vi "populateEventForceActuatorInfo.vi"(8 "error in (no error)":errorcluster, 11 "Model in":refnum<class "Model.lvclass">) -> (0 "error out":errorcluster, 3 "Model out":refnum<class "Model.lvclass">)   [LabVIEW 2016, in "Model.lvclass"]
uses:
  Model.lvclass
  Model.lvclass/Model.ctl
  ILCCommunications/ILCCommunications.lvclass/ILCCommunications.ctl
  Publisher/Publisher.lvclass/Publisher.ctl
  Common_RT_FAILC/FAILC/FAILC.lvclass/FAILC.ctl
  Common_RT_ILC/ILC/ILC.lvclass/ILC.ctl
  Common_RT_FAILC/FAILC/FAILC.lvclass
  D:/Code/ts_M1M3Support/Common_RT_ILC/ILC/ILC.lvclass
  Common_RT_ILC/ILC/ILC.lvclass
  ILCCommunications/ILCCommunications.lvclass
  Publisher/Publisher.lvclass
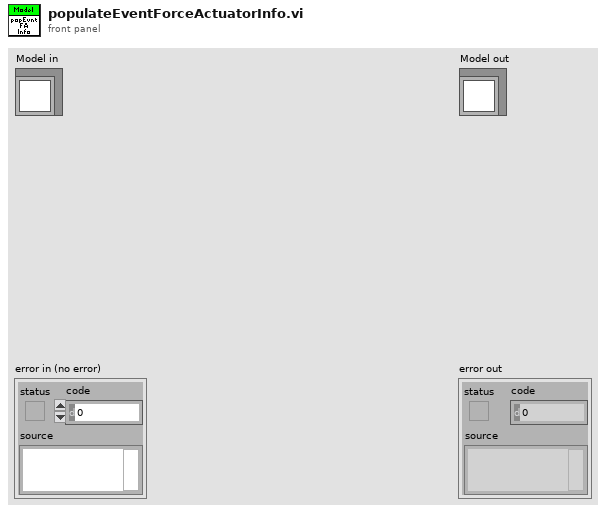
[diagram p1: front panel]
types:
  T1 = typedef "RTILC.lvlib/ILCData.ctl" = cluster{"Constants":T2, "Command":T3, "Telemetry":T5, "Responses":T6, "Timestamps":T8, "Timings":T9}
  T2 = typedef "RTILC.lvlib/ILCConstants.ctl" = cluster{"Subnet":u8, "Address":u8}
  T3 = typedef "RTILC.lvlib/ILCCommand.ctl" = cluster{"Mode":u16, "TemporaryAddress":u8, "ADCScanRate":T4, "ADCChannel":u8, "ADCOffset":sgl, "ADCSensitivity":sgl}
  T4 = typedef "RTILC.lvlib/ILCScanRates.ctl" = u8
  T5 = typedef "RTILC.lvlib/ILCTelemetry.ctl" = cluster{"UniqueID":u64, "FirmwareType":u8, "NetworkNodeType":u8, "ILCOption":u8, "NetworkNodeOption":u8, "MajorRevision":u8, "MinorRevision":u8, "FirmwareName":string, "Mode":u16, "MajorFault":bool, "MinorFault":bool, "FaultOverride":bool, "MainCalibrationError":bool, "BackupCalibrationError":bool, "UniqueIDCRCMismatch":bool, "AppTypeNodeTypeMismatch":bool, "AppMissing":bool, "AppCRCMismatch":bool, "TEDSNotFound":bool, "TEDS1Mismatch":bool, "TEDS2Mismatch":bool, "WatchdogResetDetected":bool, "BrownoutDetected":bool, "EventTrapResetDetected":bool, "MotorPowerFault":bool, "SSRPowerFault":bool, "AuxPowerFault":bool, "SMCPowerFault":bool, "TemporaryAddress":u8, "ADCScanRate":T4, "MainADCCalibrationK":sgl[], "MainSensorOffset":sgl[], "MainSensorSensitivity":sgl[], "BackupADCCalibrationK":sgl[], "BackupSensorOffset":sgl[], "BackupSensorSensitivity":sgl[]}
  T6 = typedef "RTILC.lvlib/ILCResponses.ctl" = cluster{"ReportServerID":T7, "ReportServerStatus":T7, "Mode":T7, "TemporaryAddress":T7, "Reset":T7, "ADCScanRate":T7, "ADCOffsetSensitivity":T7, "ReportCalibrationData":T7}
  T7 = typedef "RTModbus.lvlib/ExceptionCodes.ctl" = u16
  T8 = typedef "RTILC.lvlib/ILCTimestamps.ctl" = cluster{"ReportServerID":dbl, "ReportServerStatus":dbl, "Mode":dbl, "TemporaryAddress":dbl, "Reset":dbl, "ADCScanRate":dbl, "ADCOffsetSensitivity":dbl, "ReportCalibrationData":dbl}
  T9 = typedef "RTILC.lvlib/ILCTimings.ctl" = cluster{"ReportServerID":u32, "ReportServerStatus":u32, "Mode":u32, "TemporaryAddress":u32, "Reset":u32, "ADCScanRate":u32, "ADCOffsetSensitivity":u32, "ReportCalibrationData":u32}
  T10 = typedef "RTFAILC.lvlib/FAData.ctl" = cluster{"Constants":T11, "Command":T13, "Telemetry":T14, "Responses":T15, "Timings":T16, "Timestamps":T17}
  T11 = typedef "RTFAILC.lvlib/FAConstants.ctl" = cluster{"ID":i16, "Type":T12, "XPosition":sgl, "YPosition":sgl, "ZPosition":sgl}
  T12 = typedef "RTFAILC.lvlib/FATypes.ctl" = enum16{"SingleAxis", "DualAxis"}
  T13 = typedef "RTFAILC.lvlib/FACommand.ctl" = cluster{"AxialSetPoint":i32, "LateralSetPoint":i32, "AxialBoosterValveGain":sgl, "LateralBoosterValveGain":sgl}
  T14 = typedef "RTFAILC.lvlib/FATelemetry.ctl" = cluster{"ILCFault":bool, "DCAFault":bool, "BroadcastCounter":u8, "AxialLoadCellForce":sgl, "LateralLoadCellForce":sgl, "AxialBoosterValveGain":sgl, "LateralBoosterValveGain":sgl}
  T15 = typedef "RTFAILC.lvlib/FAResponses.ctl" = cluster{"BoosterValveGain":T7, "ReadBoosterValveGain":T7, "SetForce":T7, "ForceAndStatus":T7}
  T16 = typedef "RTFAILC.lvlib/FATimings.ctl" = cluster{"BroadcastSetForce":u32, "BoosterValveGain":u32, "FreezeSensorValues":u32, "ForceAndStatus":u32, "ReadBoosterValveGain":u32, "SetForce":u32}
  T17 = typedef "RTFAILC.lvlib/FATimestamps.ctl" = cluster{"BroadcastSetForce":dbl, "BoosterValveGain":dbl, "FreezeSensorValues":dbl, "ForceAndStatus":dbl, "ReadBoosterValveGain":dbl, "SetForce":dbl}
  T18 = typedef "M1M3SupportTopics.lvlib/Timestamp.ctl" = dbl
  T19 = typedef "M1M3SupportTopics.lvlib/EventForceActuatorInfo.ctl" = cluster{"Timestamp":T18, "ReferenceId":i32[], "XPosition":sgl[], "YPosition":sgl[], "ZPosition":sgl[], "ILCUniqueId":i64[], "ILCApplicationType":u8[], "NetworkNodeType":u8[], "ILCSelectedOptions":u8[], "NetworkNodeOptions":u8[], "MajorRevision":u8[], "MinorRevision":u8[], "ADCScanRate":u8[], "MainADCCalibrationK1":sgl[], "MainADCCalibrationK2":sgl[], "MainADCCalibrationK3":sgl[], "MainADCCalibrationK4":sgl[], "MainAxialLoadCellOffset":sgl[], "MainLateralLoadCellOffset":sgl[], "MainAxialLoadCellSensitivity":sgl[], "MainLateralLoadCellSensitivity":sgl[], "BackupADCCalibrationK1":sgl[], "BackupADCCalibrationK2":sgl[], "BackupADCCalibrationK3":sgl[], "BackupADCCalibrationK4":sgl[], "BackupAxialLoadCellOffset":sgl[], "BackupLateralLoadCellOffset":sgl[], "BackupAxialLoadCellSensitivity":sgl[], "BackupLateralLoadCellSensitivity":sgl[], "DCAAxialGain":sgl[], "DCALateralGain":sgl[], "DCAUniqueId":i64[], "DCAFirmwareType":u8[], "DCAMajorRevision":u8[], "DCAMinorRevision":u8[], "MainCalibrationError":bool[], "BackupCalibrationError":bool[], "DCAFirmwareUpdate":bool[], "UniqueIdCRCError":bool[], "ApplicationTypeMismatch":bool[], "ApplicationMissing":bool[], "ApplicationCRCMismatch":bool[], "OneWireMissing":bool[], "OneWire1Mismatch":bool[], "OneWire2Mismatch":bool[], "DCAUniqueIdCRCError":bool[], "DCAMainCalibrationError":bool[], "DCABackupCalibrationError":bool[], "DCAApplicationMissing":bool[], "DCAApplicationCRCMismatch":bool[], "DCABootloaderActive":bool[]}
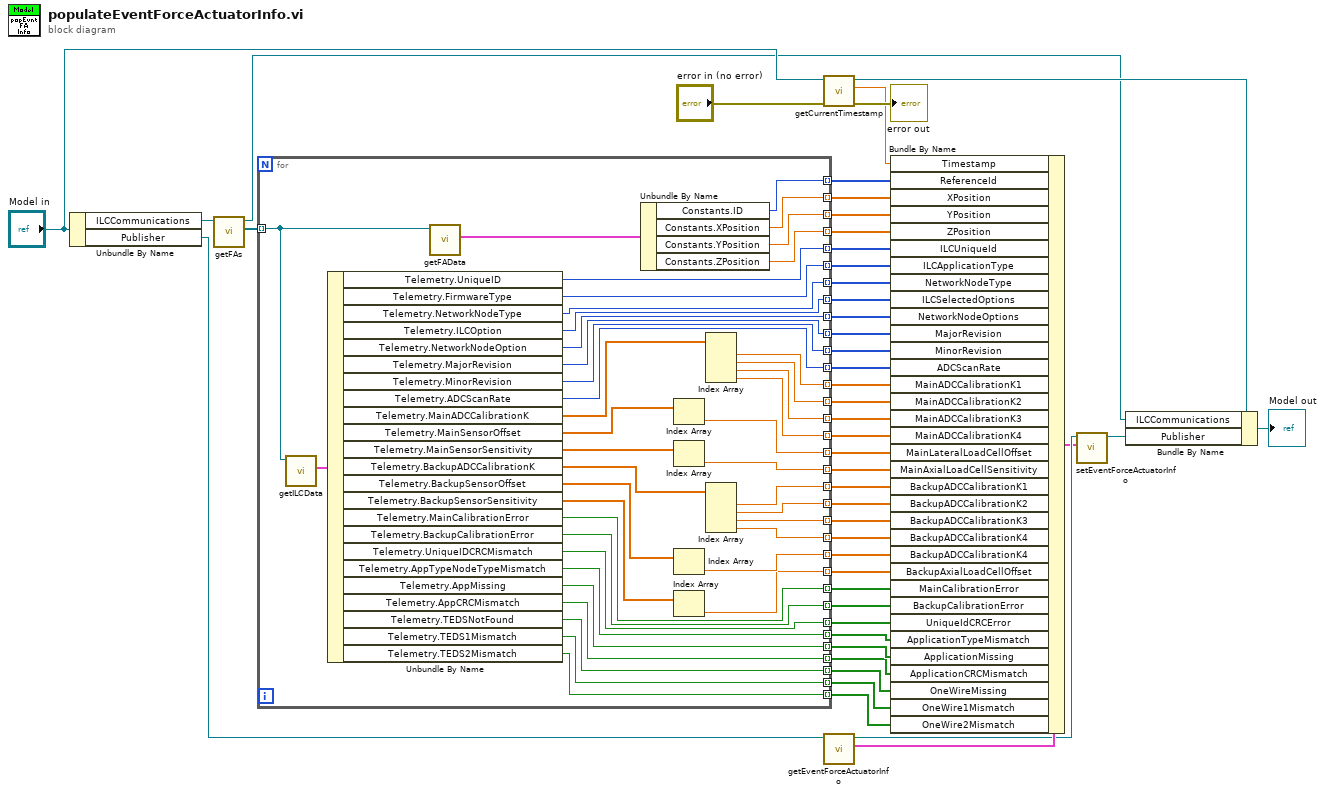
[diagram p0: block diagram]
diagram:
  n1 = Unbundle By Name("Model in") -> ("ILCCommunications"=w8:refnum<class "ILCCommunications.lvclass">, "Publisher"=w5:refnum<class "Publisher.lvclass">)
  n2 = call "getFAs.vi"("ILCCommunications in"=w8) -> ("FAs"=w6:refnum<class "FAILC.lvclass">[], "ILCCommunications out"=w7:refnum<class "ILCCommunications.lvclass">)  [unwired: 9 in]
  n3 = for {
    tunnel: w6 -> [w49] mode=indexing
    tunnel: [w87] -> w46 mode=indexing
    tunnel: [w86] -> w45 mode=indexing
    tunnel: [w85] -> w44 mode=indexing
    tunnel: [w84] -> w43 mode=indexing
    tunnel: [w83] -> w42 mode=indexing
    tunnel: [w82] -> w41 mode=indexing
    tunnel: [w81] -> w40 mode=indexing
    tunnel: [w80] -> w39 mode=indexing
    tunnel: [w79] -> w38 mode=indexing
    tunnel: [w78] -> w37 mode=indexing
    tunnel: [w77] -> w36 mode=indexing
    tunnel: [w76] -> w35 mode=indexing
    tunnel: [w74] -> w34 mode=indexing
    tunnel: [w72] -> w33 mode=indexing
    tunnel: [w70] -> w32 mode=indexing
    tunnel: [w69] -> w31 mode=indexing
    tunnel: [w68] -> w30 mode=indexing
    tunnel: [w67] -> w29 mode=indexing
    tunnel: [w65] -> w28 mode=indexing
    tunnel: [w63] -> w27 mode=indexing
    tunnel: [w62] -> w26 mode=indexing
    tunnel: [w61] -> w25 mode=indexing
    tunnel: [w60] -> w24 mode=indexing
    tunnel: [w59] -> w23 mode=indexing
    tunnel: [w58] -> w22 mode=indexing
    tunnel: [w57] -> w21 mode=indexing
    tunnel: [w56] -> w20 mode=indexing
    tunnel: [w55] -> w19 mode=indexing
    tunnel: [w54] -> w18 mode=indexing
    tunnel: [w53] -> w17 mode=indexing
    tunnel: [w52] -> w11 mode=indexing
    tunnel: [w51] -> w10 mode=indexing
    tunnel: [w50] -> w9 mode=indexing
    n4 = call "getILCData.vi"("ILC in"=w49) -> ("ILCData"=w89:T1)  [unwired: 9 in, 1 out]
    n5 = Unbundle By Name(w89) -> ("Telemetry.UniqueID"=w87:u64, "Telemetry.FirmwareType"=w86:u8, "Telemetry.NetworkNodeType"=w85:u8, "Telemetry.ILCOption"=w84:u8, "Telemetry.NetworkNodeOption"=w83:u8, "Telemetry.MajorRevision"=w82:u8, "Telemetry.MinorRevision"=w81:u8, "Telemetry.ADCScanRate"=w80:T4, "Telemetry.MainADCCalibrationK"=w88:sgl[], "Telemetry.MainSensorOffset"=w75:sgl[], "Telemetry.MainSensorSensitivity"=w73:sgl[], "Telemetry.BackupADCCalibrationK"=w71:sgl[], "Telemetry.BackupSensorOffset"=w66:sgl[], "Telemetry.BackupSensorSensitivity"=w64:sgl[], "Telemetry.MainCalibrationError"=w62:bool, "Telemetry.BackupCalibrationError"=w61:bool, "Telemetry.UniqueIDCRCMismatch"=w60:bool, "Telemetry.AppTypeNodeTypeMismatch"=w59:bool, "Telemetry.AppMissing"=w58:bool, "Telemetry.AppCRCMismatch"=w57:bool, "Telemetry.TEDSNotFound"=w56:bool, "Telemetry.TEDS1Mismatch"=w55:bool, "Telemetry.TEDS2Mismatch"=w54:bool)
    n6 = call "getFAData.vi"("FAILC in"=w49) -> ("FAData"=w48:T10)  [unwired: 9 in, 1 out]
    n7 = Unbundle By Name(w48) -> ("Constants.ID"=w53:i16, "Constants.XPosition"=w52:sgl, "Constants.YPosition"=w51:sgl, "Constants.ZPosition"=w50:sgl)
    n8 = Index Array(array=w75) -> (element=w74:sgl)  [unwired: 1 in]
    n9 = Index Array(array=w73) -> (element=w72:sgl)  [unwired: 1 in]
    n10 = Index Array(array=w66) -> (element=w65:sgl)  [unwired: 1 in]
    n11 = Index Array(array=w64) -> (element=w63:sgl)  [unwired: 1 in]
    n12 = Index Array(array=w88) -> (element #1=w79:sgl, element #2=w78:sgl, element #3=w77:sgl, element #4=w76:sgl)  [unwired: 4 in]
    n13 = Index Array(array=w71) -> (element #1=w70:sgl, element #2=w69:sgl, element #3=w68:sgl, element #4=w67:sgl)  [unwired: 4 in]
  }
  n14 = call "getCurrentTimestamp.vi"("error in (no error)"="error in (no error)", "Model in"="Model in") -> ("error out"=→"error out":errorcluster, "Timestamp"=w12:T18, "Model out"=w15:refnum<class "Model.lvclass">)  [unwired: 7 in]
  n15 = call "getEventForceActuatorInfo.vi"("Publisher in"=w5) -> ("EventForceActuatorInfo"=w4:T19, "Publisher out"=w3:refnum<class "Publisher.lvclass">)  [unwired: 9 in]
  n16 = Bundle By Name(cluster=w4, "Timestamp"=w12, "ReferenceId"=w17, "XPosition"=w11, "YPosition"=w10, "ZPosition"=w9, "ILCUniqueId"=w46, "ILCApplicationType"=w45, "NetworkNodeType"=w44, "ILCSelectedOptions"=w43, "NetworkNodeOptions"=w42, "MajorRevision"=w41, "MinorRevision"=w40, "ADCScanRate"=w39, "MainADCCalibrationK1"=w38, "MainADCCalibrationK2"=w37, "MainADCCalibrationK3"=w36, "MainADCCalibrationK4"=w35, "MainLateralLoadCellOffset"=w34, "MainAxialLoadCellSensitivity"=w33, "BackupADCCalibrationK1"=w32, "BackupADCCalibrationK2"=w31, "BackupADCCalibrationK3"=w30, "BackupADCCalibrationK4"=w29, "BackupADCCalibrationK4"=w28, "BackupAxialLoadCellOffset"=w27, "MainCalibrationError"=w26, "BackupCalibrationError"=w25, "UniqueIdCRCError"=w24, "ApplicationTypeMismatch"=w23, "ApplicationMissing"=w22, "ApplicationCRCMismatch"=w21, "OneWireMissing"=w20, "OneWire1Mismatch"=w19, "OneWire2Mismatch"=w18) -> (w1:T19)
  n17 = call "setEventForceActuatorInfo.vi"("EventForceActuatorInfo"=w1, "Publisher in"=w3) -> ("Publisher out"=w2:refnum<class "Publisher.lvclass">)  [unwired: 9 in]
  n18 = Bundle By Name(cluster=w15, "ILCCommunications"=w7, "Publisher"=w2) -> (→"Model out":refnum<class "Model.lvclass">)
